vi "崩溃文件路径.vi"() -> (3 "添加的路径":path)   [LabVIEW 2016]
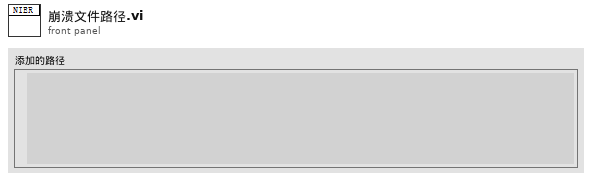
[diagram p1: front panel]
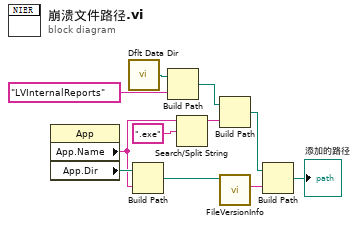
[diagram p0: block diagram]
diagram:
  n1 = property class="App"() -> ("App.Name"=w3:string, "App.Dir"=w4:path)  [unwired: 2 in, 2 out]
  n2 = call <vilib>:"Dflt Data Dir.vi"() -> ("App:Default Data Directory"=w11:path)
  n3 = Build Path(base path=w4, name or relative path=w3) -> (appended path=w2:path)
  n4 = Build Path(base path=w11, name or relative path="LVInternalReports" ("名称或相对路径")) -> (appended path=w9:path)
  n5 = Search/Split String(string=w3, search string/char (-)=".exe" ("搜索字符串/字符(-)")) -> (substring before match=w7:string)  [unwired: 1 in, 2 out]
  n6 = Build Path(base path=w9, name or relative path=w7) -> (appended path=w6:path)
  n7 = call <vilib>:"FileVersionInfo.vi"("Application Path in"=w2) -> ("File Version Info"=w1:string)  [unwired: 7 in, 3 out]
  n8 = Build Path(base path=w6, name or relative path=w1) -> (appended path=→"添加的路径":path)
